vi "TangoCalibrate.vi"(8 "error in (no error)":errorcluster, 11 "plLSID in":i32) -> (0 "error out":errorcluster, 2 "X Limits":dbl[](array[numeric]) caption="X Limits [µm]" format="%#_10f", 3 "Y Limits":dbl[](array[numeric]) caption="Y Limits [µm]" format="%#_12f")   [LabVIEW 2018, in "TangoOWN.lvlib"]
uses:
  TangoOWN.lvlib
  SDK/Tango.lvlib
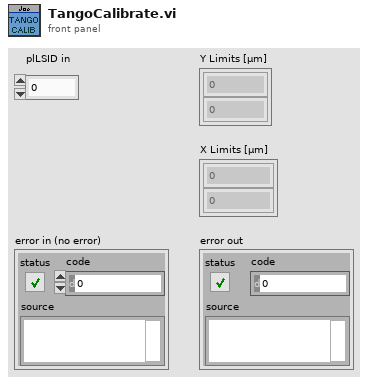
[diagram p1: front panel]
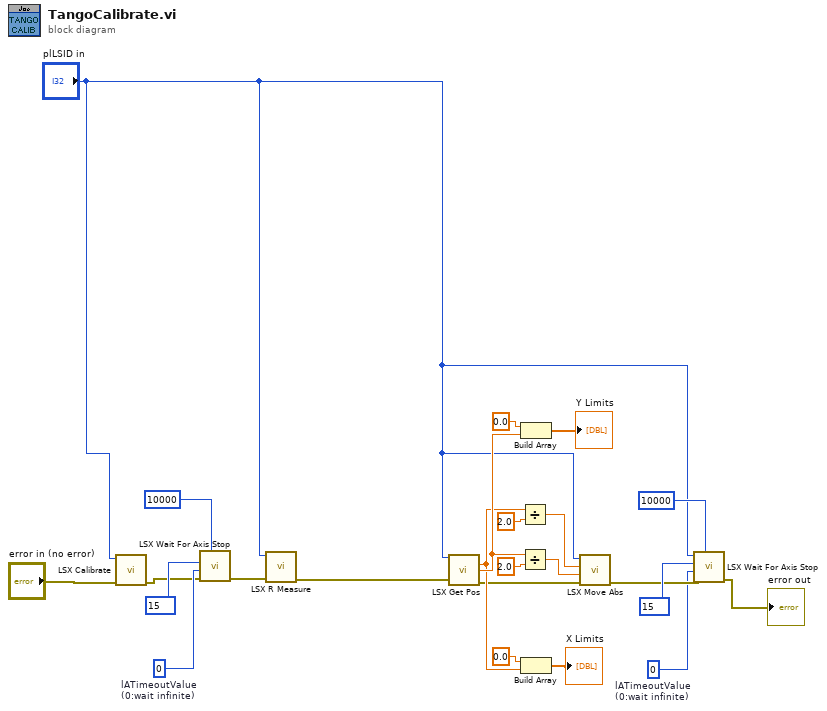
[diagram p0: block diagram]
diagram:
  w5 = 0  # lATimeoutValue (0:wait infinite)
  w8 = 0  # lATimeoutValue (0:wait infinite)
  n1 = call "LSX Calibrate.vi"("error in (no error)"="error in (no error)", "lLSID"="plLSID in") -> ("error out"=w4:errorcluster)  [unwired: 8 in, 1 out]
  n2 = call "LSX Wait For Axis Stop.vi"("pbATimeout"=10000, "error in (no error)"=w4, "lATimeoutValue"=w5, "lAFlags"=i8 15) -> ("error out"=w3:errorcluster)  [unwired: 5 in, 2 out]
  n3 = call "LSX R Measure.vi"("error in (no error)"=w3, "lLSID"="plLSID in") -> ("error out"=w1:errorcluster)  [unwired: 8 in, 1 out]
  n4 = call "LSX Get Pos.vi"("lLSID"="plLSID in", "error in (no error)"=w1) -> ("pdX out"=w22:dbl, "pdY out"=w23:dbl, "error out"=w17:errorcluster)  [unwired: 8 in, 3 out]
  n5 = Divide(x=w22, y=2.0) -> (x/y=w19:dbl)
  n6 = Divide(x=w23, y=2.0) -> (x/y=w18:dbl)
  n7 = Build Array(0.0 ("element"), w23) -> (→"Y Limits":dbl[])
  n8 = Build Array(0.0 ("element"), w22) -> (→"X Limits":dbl[])
  n9 = call "LSX Move Abs.vi"("error in (no error)"=w17, "dY"=w18, "dX"=w19, "lLSID"="plLSID in") -> ("error out"=w10:errorcluster)  [unwired: 6 in, 1 out]
  n10 = call "LSX Wait For Axis Stop.vi"("pbATimeout"=10000, "error in (no error)"=w10, "lATimeoutValue"=w8, "lAFlags"=i8 15, "lLSID"="plLSID in") -> ("error out"=→"error out":errorcluster)  [unwired: 4 in, 2 out]
